vi "read-cluster-tag-name.vi"(8 "error in (no error)":errorcluster, 11 "dbc in":refnum<class "dbc.lvclass">) -> (0 "error out":errorcluster, 2 "tag.cluster":string, 3 "dbc out":refnum<class "dbc.lvclass">)   [LabVIEW 2015, in "dbc.lvclass"]
uses:
  dbc.lvclass
  dbc.lvclass/dbc.ctl
  read-tree-ref.vi
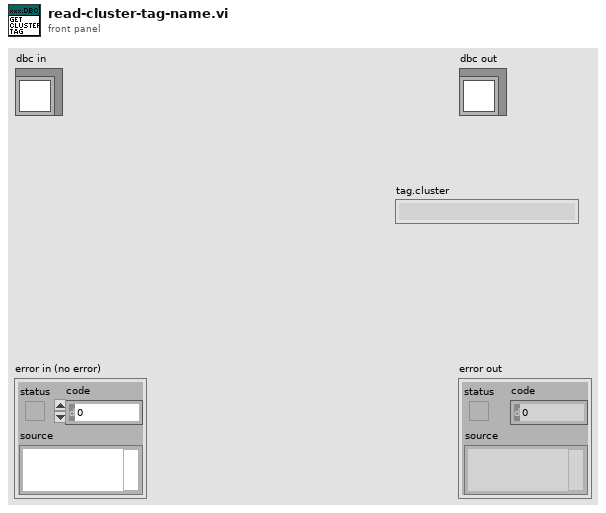
[diagram p1: front panel]
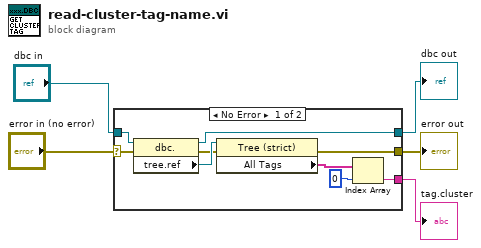
[diagram p0: block diagram]
diagram:
  n1 = case shown="No Error" "error in (no error)" {
    selector: "error in (no error)" -> [w7 w16]
    tunnel: [w6 w16] -> w4
    tunnel: [w13 w15] -> w2
    tunnel: "dbc in" -> [w14 w15]
    tunnel: [w9 _] -> w1
    frame No Error {
      n2 = property class="dbc."(reference=w14, error in=w7) -> (reference out=w13:refnum<class "dbc.lvclass">, error out=w8:errorcluster, "tree.ref"=w12:refnum<vi>)
      n3 = property class="Tree (strict)"(reference=w12, error in=w8) -> (error out=w6:errorcluster, "All Tags"=w11:string[])  [unwired: 1 out]
      n4 = Index Array(array=w11, index=0) -> (element=w9:string)
    }
    frame Error {
    }
  }
  "error out" <- w4
  "dbc out" <- w2
  "tag.cluster" <- w1
